vi "Config-Diagnostics.vi"(8 "error in (no error)":errorcluster, 11 "Refnum in":T2) -> (0 "error out":errorcluster, 2 "Diagnostics":T1, 3 "Refnum out":T2)   [LabVIEW 2021, in "UDP_Config.lvclass"]
uses:
  UDP_Config.lvclass
  <vilib>/Utility/config.llb/Config Data RefNum.ctl
  Diagnostics.ctl
  <vilib>/Utility/config.llb/Read Key (Boolean).vi
  <vilib>/Utility/config.llb/Read Key (String).vi
  <vilib>/Utility/config.llb/NI_LVConfig.lvlib
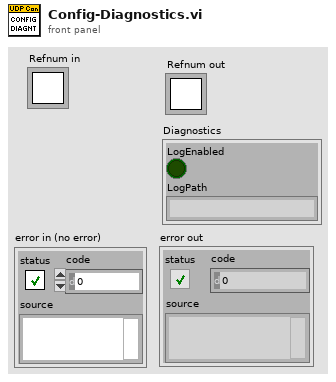
[diagram p1: front panel]
types:
  T1 = typedef "Diagnostics.ctl" = cluster{"LogEnabled":bool, "LogPath":string}
  T2 = typedef "NI_LVConfig.lvlib/Config Data RefNum.ctl" = refnum<k1>
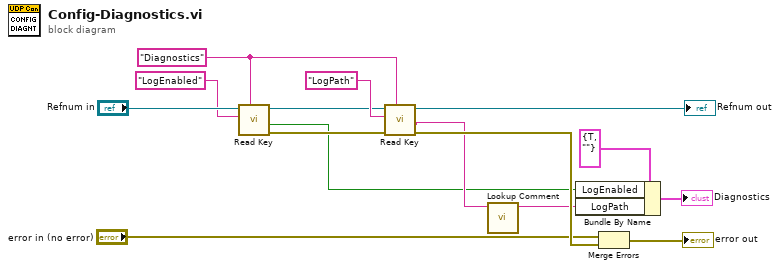
[diagram p0: block diagram]
diagram:
  w12 = "Diagnostics" ("key")
  n1 = call-poly <vilib>:"Read Key.vi"("section"=w12, "key"="LogEnabled", "refnum"="Refnum in") -> ("error out"=w13:errorcluster, "value"=w2:bool, "refnum out"=w9:T2)  [unwired: 5 in, 1 out]
  n2 = call-poly <vilib>:"Read Key.vi"("section"=w12, "error in (no error)"=w13, "key"="LogPath", "refnum"=w9) -> ("error out"=w14:errorcluster, "value"=w5:string, "refnum out"=→"Refnum out":T2)  [unwired: 4 in, 1 out]
  n3 = call "Lookup Comment.vi"("String in"=w5) -> ("Value"=w3:string)  [unwired: 3 in, 1 out]
  n4 = Bundle By Name(cluster=T1 {"LogEnabled"=TRUE, "LogPath"=""} ("Diagnostics"), "LogEnabled"=w2, "LogPath"=w3) -> (→"Diagnostics":T1)
  n5 = Merge Errors("error in (no error)", w14) -> (→"error out":errorcluster)
